vi "sub_AO-gen.vi"(8 "error in (no error)":errorcluster, 11 "level":bool) -> (0 "error out":errorcluster)   [LabVIEW 2019]
uses:
  _ctrl/init-w-close.ctl
  cmd_timecheck.ctl
panel:
  out "Array":errorcluster[](array[cluster])
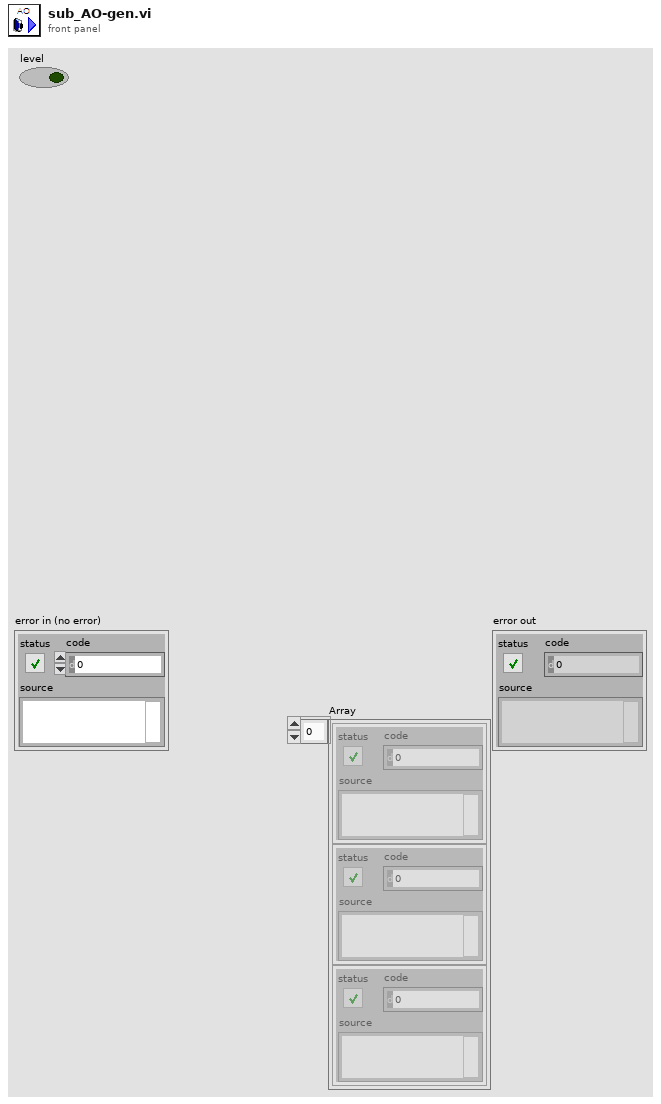
[diagram p1: front panel]
types:
  T1 = typedef "cmd_timecheck.ctl" = enum16{"Group start", "Group end", "Grout dt", "Ch start", "Ch end", "Ch dt", "init", "NF start", "NF stop", "idrc start", "idrc stop", "scope start", "scope stop", "ao start", "ao stop", "relay start", "relay stop", "NF read start", "NF read stop", "NF set start", "NF set stop", "idrc level start", "idrc level stop", "scope trig start", "scope trig stop", "relay dischar star", "relay dischar stop", "data process start", "data process stop", "ch-relay on start", "ch-relay on stop", "hw set start", "hw set stop", "pwr-in on start", "pwr-in on stop", "pwr-out on start", "pwr-out on stop", "ao on start", "ao on stop", "ao 0v start", "ao 0v stop", "pwr-in off start", "pwr-in off stop", "relay-all off start", "relay-all off stop", "pwr-out off start", "pwr-out off stop", "discharge start", "discharge stop", "950 read start", "950 read stop"}
  T2 = typedef "init-w-close.ctl" = enum16{"open", "init", "write", "close"}
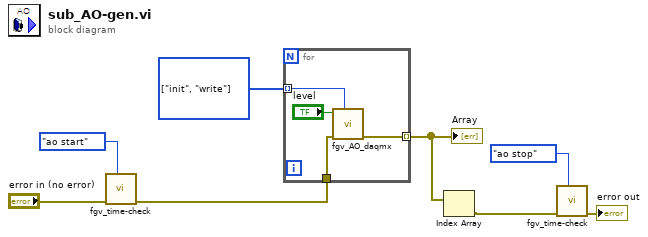
[diagram p0: block diagram]
diagram:
  w8 = T2[] [enum."init", enum."write"] items=["open", "init", "write", "close"]
  n1 = call "fgv_time-check.vi"("cmd"=cmd_timecheck."ao start", "error in (no error)"="error in (no error)") -> ("error out"=w6:errorcluster)  [unwired: 8 in, 1 out]
  n2 = for {
    tunnel: w8 -> [w12] mode=indexing
    tunnel: [w11] -> w4 mode=indexing
    tunnel: w6 -> [w10]
    n3 = call "fgv_AO_daqmx.vi"("cmd"=w12, "error in"=w10, "level"="level") -> ("error out"=w11:errorcluster)  [unwired: 8 in]
  }
  "Array" <- w4
  n4 = Index Array(array=w4) -> (element=w3:errorcluster)  [unwired: 1 in]
  n5 = call "fgv_time-check.vi"("cmd"=cmd_timecheck."ao stop", "error in (no error)"=w3) -> ("error out"=→"error out":errorcluster)  [unwired: 8 in, 1 out]
